vi "Example FroLoop Tunnel 1.vi"(8 "Error In":errorcluster) -> (0 "Error Out":errorcluster, 3 "ind1":i32[](array[numeric]))   [LabVIEW 2014]
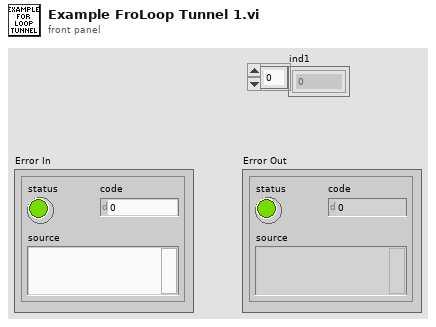
[diagram p1: front panel]
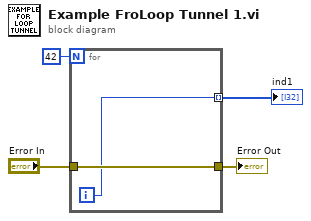
[diagram p0: block diagram]
diagram:
  n1 = for {
    N: 42 -> [_]
    tunnel: "Error In" -> [w6]
    tunnel: [w6] -> w3
    tunnel: [w5] -> w2 mode=indexing
    i -> [w5]
  }
  "Error Out" <- w3
  "ind1" <- w2
